vi "Open TCPIP Port V.vi"(8 "error in (no error)":errorcluster, 10 "IPAddr":string, 11 "tcpPort":string) -> (0 "error out":errorcluster, 3 "function return":i16)   [LabVIEW 2009, in "VantagePro.lvlib"]
doc: "DllAccess short int _stdcall OpenTCPIPPort_V (const char *tcpPort, const char *IPAddr);"
uses:
  VantagePro.lvlib
  <userlib>/VantagePro/VantagePro.dll
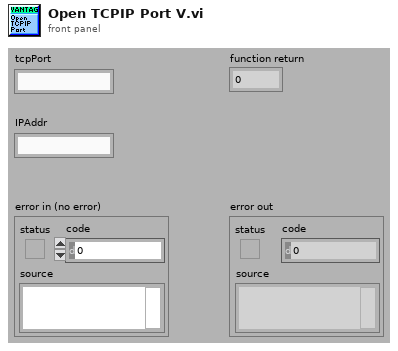
[diagram p1: front panel]
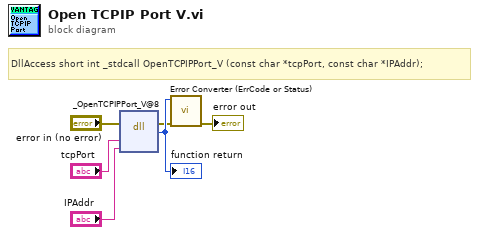
[diagram p0: block diagram]
diagram:
  # "DllAccess short int _stdcall OpenTCPIPPort_V (const char *tcpPort, const char *IPAddr);"
  n1 = dll-call lib="C:/Program Files/National Instruments/LabVIEW 2010/user.lib/VantagePro/VantagePro.*" fn="_OpenTCPIPPort_V@8"(error in="error in (no error)", "tcpPort"="tcpPort", "IPAddr"="IPAddr") -> (error out=w2:errorcluster, w6:i16)  [unwired: 4 in, 1 out]
  "function return" <- w6
  n2 = call "Error Converter (ErrCode or Status).vi"("error in (no error)"=w2, "error code"=w6) -> ("error out"=→"error out":errorcluster)  [unwired: 9 in]
